vi "idxArrayToBoolArray.vi"(8 "error in (no error)":errorcluster, 9 "Idx Array":i32[](array[numeric]), 10 "Length of Bool Array":i32, 11 "MatOper in":refnum<class "MatOper.lvclass">) -> (0 "error out":errorcluster, 2 "Bool Array":bool[](array[boolean]), 3 "MatOper out":refnum<class "MatOper.lvclass">)   [LabVIEW 2016, in "OfcFunc.lvlib" / "MatOper.lvclass"]
doc: "Translate the index array to boolean array. (e.g. [0, 2] -> [T, F, T])."
uses:
  MatOper.lvclass
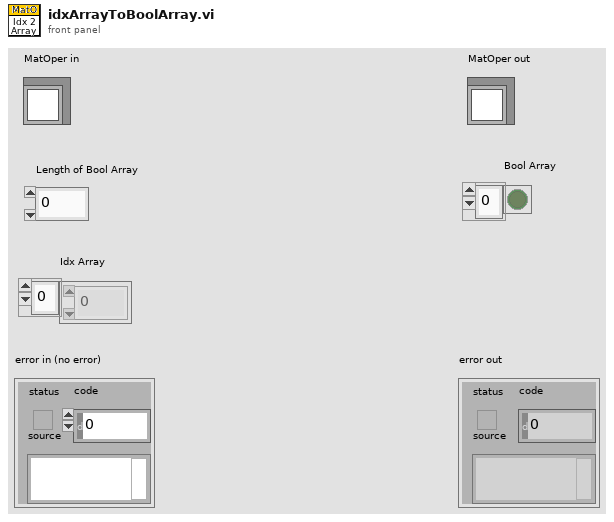
[diagram p1: front panel]
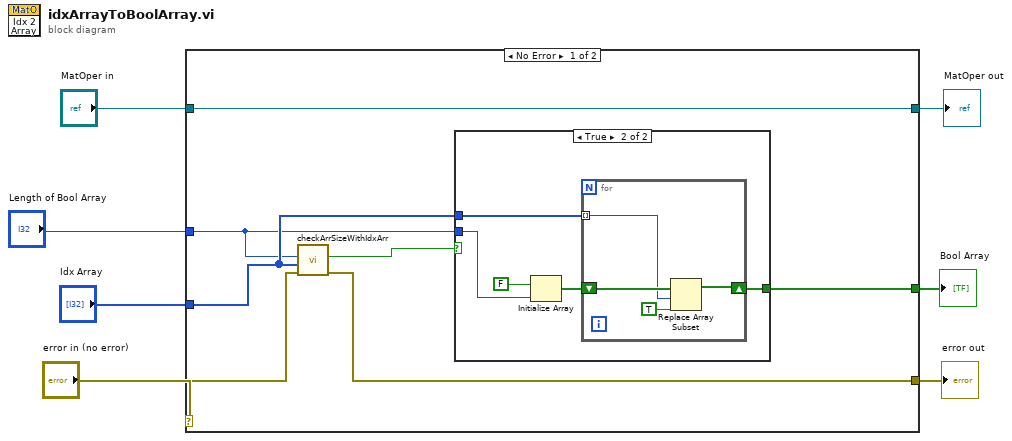
[diagram p0: block diagram]
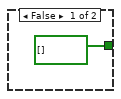
[diagram p2: hidden frame]
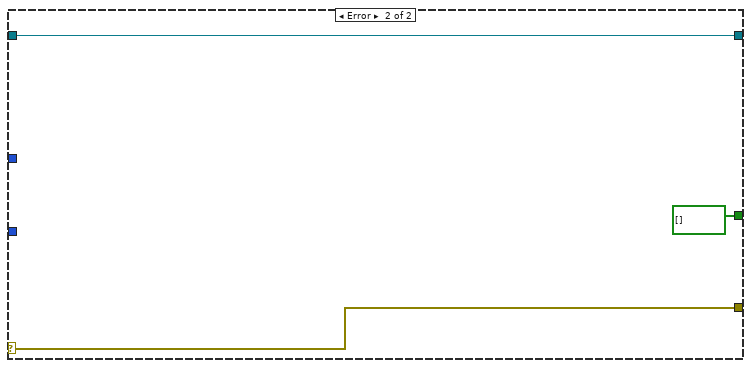
[diagram p3: hidden frame]
diagram:
  n1 = case shown="No Error" "error in (no error)" {
    selector: "error in (no error)" -> [w9 w27]
    tunnel: [w8 w27] -> w6
    tunnel: [w14 w26] -> w4
    tunnel: "MatOper in" -> [w14 w26]
    tunnel: [w12 bool[] []] -> w3
    tunnel: "Idx Array" -> [w11 _]
    tunnel: "Length of Bool Array" -> [w10 _]
    frame No Error {
      n2 = call "checkArrSizeWithIdxArr.vi"("error in (no error)"=w9, "Idx Array"=w11, "Array Size"=w10) -> ("error out"=w8:errorcluster, "In Spec"=w13:bool)  [unwired: 6 in, 1 out]
      n3 = case shown="True" w13 {
        tunnel: [bool[] [] w18] -> w12
        tunnel: w10 -> [_ w17]
        tunnel: w11 -> [_ w16]
        frame False {
        }
        frame True {
          n4 = Initialize Array(FALSE, w17) -> (w19:bool[])
          n5 = for {
            shift-right: [w22] -> w18
            shift-left: w19 -> [w24]
            tunnel: w16 -> [w23] mode=indexing
            n6 = Replace Array Subset(array=w24, new element=TRUE, index=w23) -> (w22:bool[])
          }
        }
      }
    }
    frame Error {
    }
  }
  "error out" <- w6
  "MatOper out" <- w4
  "Bool Array" <- w3
